vi "Populate_Do.vi"(8 "error in (no error)":errorcluster, 9 "Value":string, 10 "Lower case name":string, 11 "Caraya Unit Test in":refnum<class "Caraya Test.lvclass">) -> (0 "error out":errorcluster, 1 "Success?":bool, 3 "Caraya Unit Test out":refnum<class "Caraya Test.lvclass">)   [LabVIEW 2020, in "ProjectBuilder.lvlib" / "Caraya Test.lvclass"]
doc: "Override to populate private data from strings.\n\nSee action documentation for populate description."
uses:
  Caraya Test.lvclass
  Caraya Test.lvclass/Caraya Test.ctl
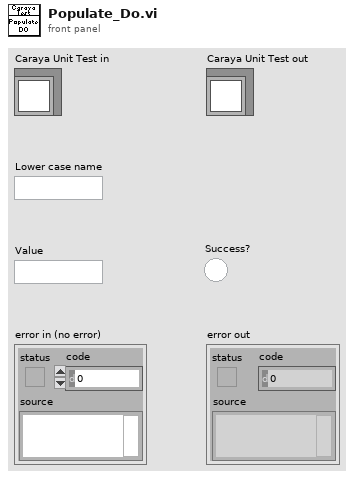
[diagram p1: front panel]
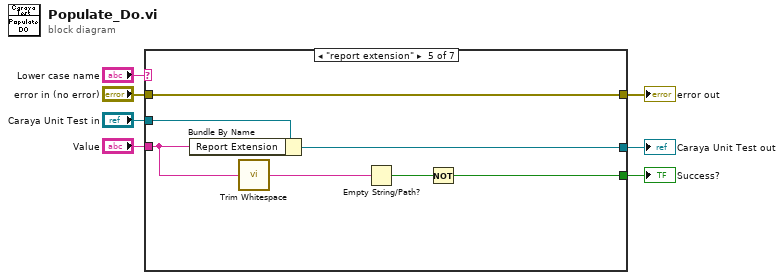
[diagram p0: block diagram]
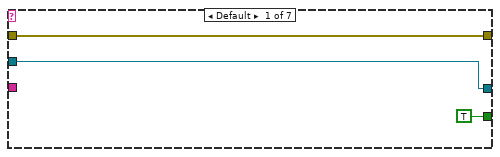
[diagram p2: hidden frame]
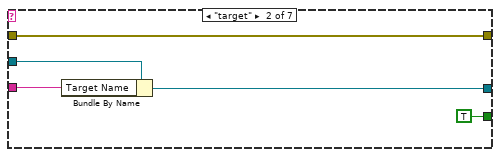
[diagram p3: hidden frame]
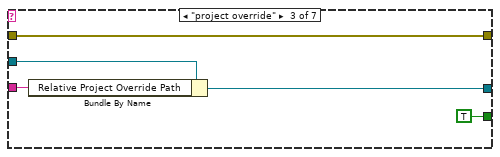
[diagram p4: hidden frame]
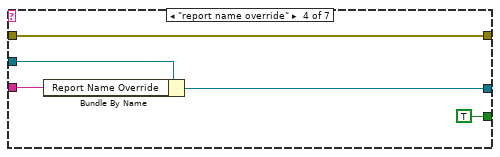
[diagram p5: hidden frame]
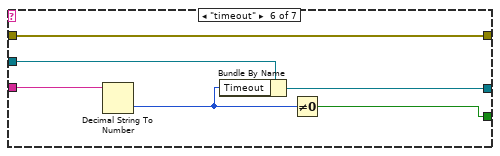
[diagram p6: hidden frame]
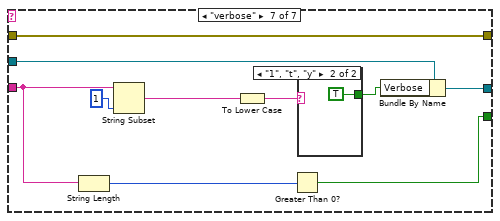
[diagram p7: hidden frame]
diagram:
  n1 = case shown="\"report extension\"" "Lower case name" {
    tunnel: [TRUE TRUE TRUE TRUE w27 w34 w39] -> w3
    tunnel: [w9 w14 w19 w24 w31 w37 w47] -> w2
    tunnel: "Caraya Unit Test in" -> [w9 w15 w20 w25 w32 w38 w48]
    tunnel: [w8 w12 w17 w22 w30 w36 w46] -> w1
    tunnel: "error in (no error)" -> [w8 w12 w17 w22 w30 w36 w46]
    tunnel: "Value" -> [_ w13 w18 w23 w29 w35 w41]
    frame Default {
    }
    frame "target" {
      n2 = Bundle By Name(cluster=w15, "Target Name"=w13) -> (w14:refnum<class "Caraya Test.lvclass">)
    }
    frame "project override" {
      n3 = Bundle By Name(cluster=w20, "Relative Project Override Path"=w18) -> (w19:refnum<class "Caraya Test.lvclass">)
    }
    frame "report name override" {
      n4 = Bundle By Name(cluster=w25, "Report Name Override"=w23) -> (w24:refnum<class "Caraya Test.lvclass">)
    }
    frame "report extension" {
      n5 = Bundle By Name(cluster=w32, "Report Extension"=w29) -> (w31:refnum<class "Caraya Test.lvclass">)
      n6 = call <vilib>:"Trim Whitespace.vi"("string"=w29) -> ("trimmed string"=w26:string)  [unwired: 1 in]
      n7 = Empty String/Path?(string/path=w26) -> (empty?=w28:bool)
      n8 = Not(x=w28) -> (.not. x?=w27:bool)
    }
    frame "timeout" {
      n9 = Decimal String To Number(string=w35) -> (number=w33:i32)  [unwired: 2 in, 1 out]
      n10 = Bundle By Name(cluster=w38, "Timeout"=w33) -> (w37:refnum<class "Caraya Test.lvclass">)
      n11 = Not Equal To 0?(x=w33) -> (x != 0?=w34:bool)
    }
    frame "verbose" {
      n12 = String Length(string=w41) -> (length=w40:i32)
      n13 = String Subset(string=w41, length (rest)=1 ("length (rest)")) -> (substring=w44:string)  [unwired: 1 in]
      n14 = To Lower Case(string=w44) -> (all lower case string=w43:string)
      n15 = Greater Than 0?(x=w40) -> (x > 0?=w39:bool)
      n16 = case shown="\"1\", \"t\", \"y\"" w43 {
        tunnel: [_ TRUE] -> w42
        frame Default {
        }
        frame "1", "t", "y" {
        }
      }
      n17 = Bundle By Name(cluster=w48, "Verbose"=w42) -> (w47:refnum<class "Caraya Test.lvclass">)
    }
  }
  "error out" <- w1
  "Caraya Unit Test out" <- w2
  "Success?" <- w3
